vi "Read Initialized.vi"(11 "Interlock in":refnum<class "Interlock.lvclass">) -> (2 "Initialized":bool, 3 "Interlock out":refnum<class "Interlock.lvclass">)   [LabVIEW 2015, in "Interlocks.lvlib" / "Interlock.lvclass"]
uses:
  Interlock.lvclass
  Interlock.lvclass/Interlock.ctl
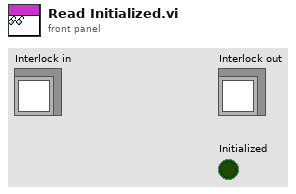
[diagram p1: front panel]
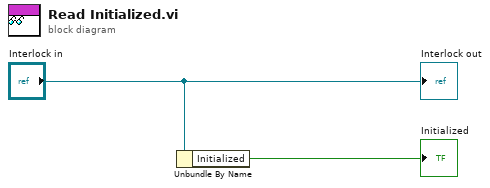
[diagram p0: block diagram]
diagram:
  n1 = Unbundle By Name("Interlock in") -> ("Initialized"=→"Initialized":bool)
  "Interlock out" <- "Interlock in"
